vi "Close Device.vi"(8 "error in (no error)":errorcluster, 11 "Topas4 in":refnum<class "Topas4.lvclass">) -> (0 "error out":errorcluster, 3 "Topas4 out":refnum<class "Topas4.lvclass">)   [LabVIEW 2020, in "Topas4.lvclass"]
uses:
  Topas4.lvclass
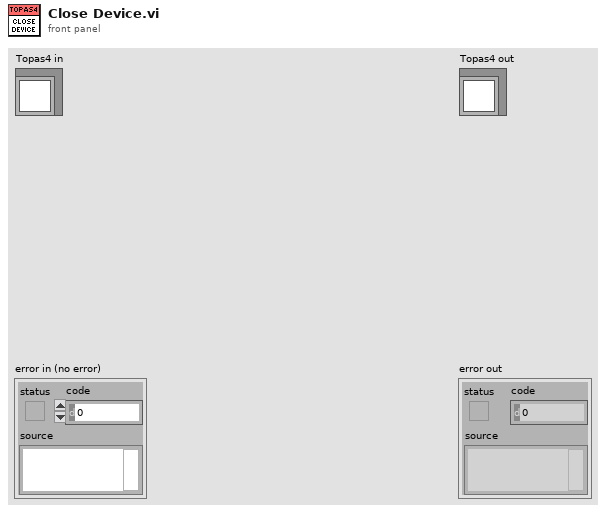
[diagram p1: front panel]
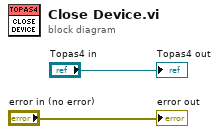
[diagram p0: block diagram]
diagram:
  "error out" <- "error in (no error)"
  "Topas4 out" <- "Topas4 in"
